vi "WhileLoop.vi"() -> ()   [LabVIEW 2019]
panel:
  out "Iterator":i32
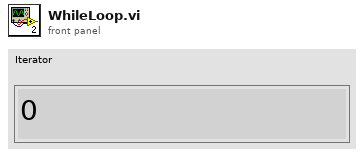
[diagram p1: front panel]
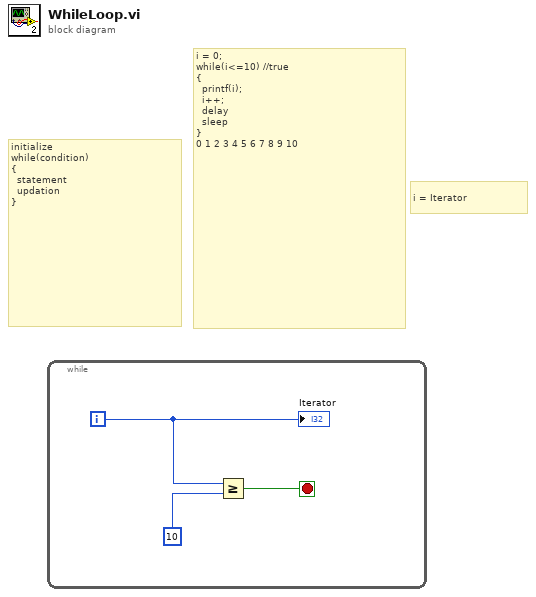
[diagram p0: block diagram]
diagram:
  # "i = Iterator"
  # "i = 0;\nwhile(i<=10) //true\n{\n  printf(i);\n  i++;\n  delay\n  sleep\n}\n0 1 2 3 4 5 6 7 8 9 10"
  # "initialize\nwhile(condition)\n{\n  statement\n  updation\n}"
  n1 = while {
    i -> [w3]
    stop <- w1 stop-if-true
    n2 = Greater Or Equal?(x=w3, y=10) -> (x >= y?=w1:bool)
    "Iterator" <- w3
  }
